vi "getData.vi"() -> ()   [LabVIEW 2014]
uses:
  <vilib>/FPGAPlugInAG/cRIO-9066/niLvFpga_Open_cRIO-9066.vi
  <vilib>/rvi/errors/niLvFpgaMergeErrorWithErrorCode.vi
  <vilib>/Utility/file.llb/Write To Spreadsheet File (DBL).vi
  <vilib>/FPGAPlugInAG/cRIO-9066/niLvFpga_Close_cRIO-9066.vi
  <vilib>/rvi/interface/nirviOpenFPGA/nirviOpenFPGA.xnode
  FPGA Bitfiles/forcecontroledu_FPGATarget_impElbow_wp9Tcc+MyeY.lvbitx
  FPGA VIs/imp_Elbow.vi
  <vilib>/rvi/interface/nirviMethod/nirviMethod.xnode
  <vilib>/rvi/interface/nirviCloseFPGA/nirviCloseFPGA.xnode
  <vilib>/FPGAPlugInAG/cRIO-9066/niLvFpga_ReadFifo_cRIO-9066.vi
panel:
  out "Loop count":i32=10000
  out "FIFO empty":bool
  out "sampling time":u32=10000
  out "message":string=" INSTRUCTIONS:\r\rNormal Use:  When using subVIs that incorporate the error in/error out (or error I/O) structure, place this handler where you want to inform the user of an error, typically at the end of the I/O data path, as the last action of the program.  If the error in error? is ERROR, the handler creates a message describing the error and its source.  If the type of dialog = 1 (default), the message is displayed to the user, who can only acknowedge it.  If the type = 2, the user can acknowledge the message or abort execution; aborting a program with active I/O is not recommended.  If the type = 0, no message is displayed; this is used to process the error programmatically, and the error out cluster elements are wired to individual terminals for that reason.  \r\rOther Use:\n\r\nlocal testing.  To test the error code of a subVI or function that does not have the error I/O structure, you can wire its error code and a source string to the local error code and error source inputs.  If error in error? indicates no error and error code is not equal to 0, the local code and source are substituted for the error in values, and error? is set TRUE (ERROR)."
  out "Elements Remaining":u32=10000
  in  "Number of samples":i32=10000
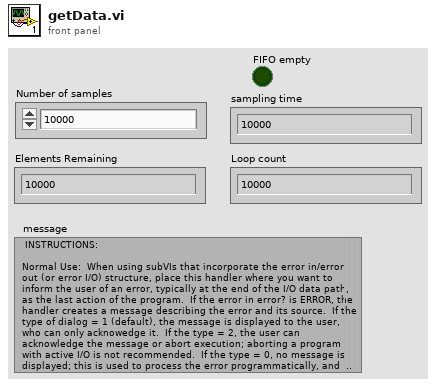
[diagram p1: front panel]
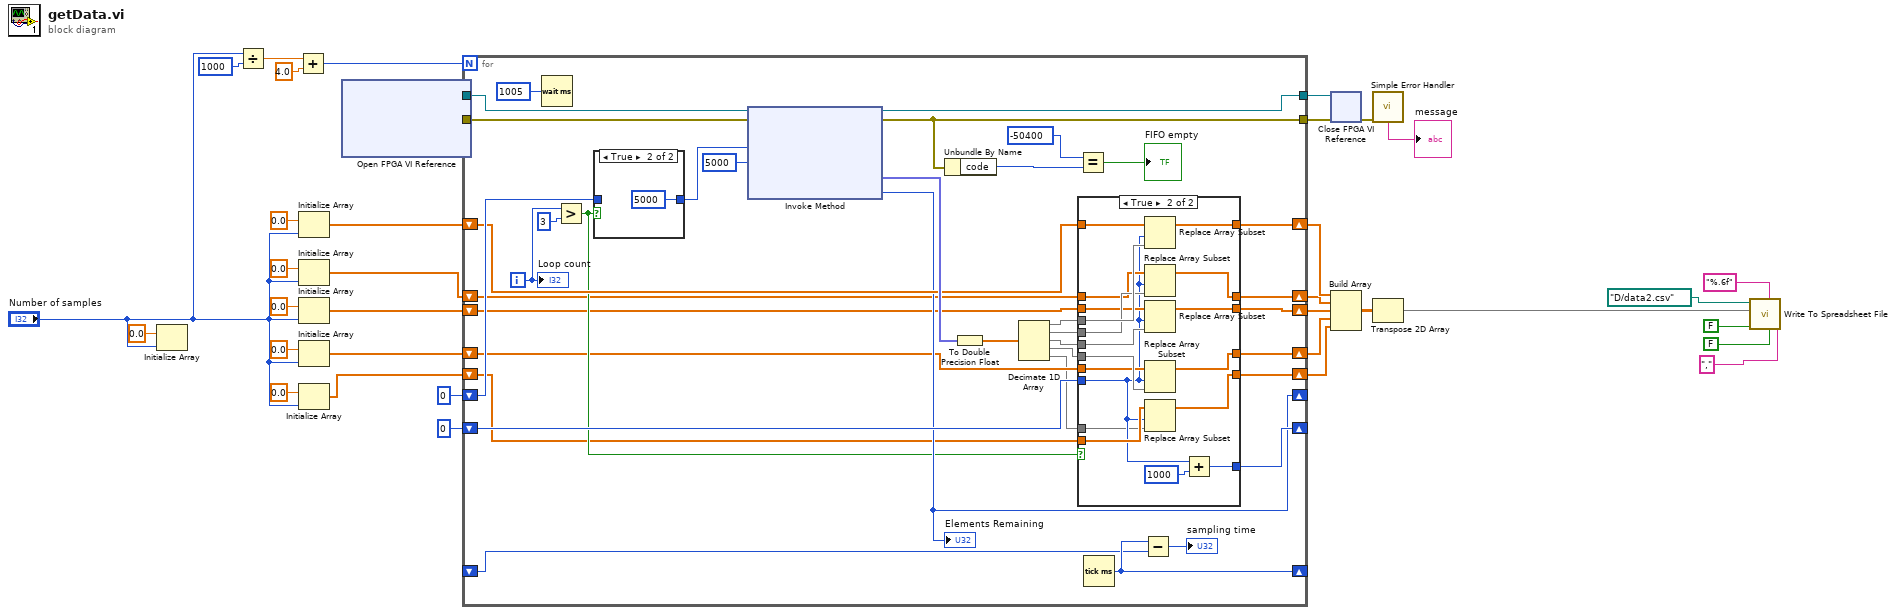
[diagram p0: block diagram]
diagram:
  n1 = Initialize Array(0.0 ("element"), "Number of samples") -> ()  [unwired: 1 out]
  n2 = Divide(x="Number of samples", y=1000) -> (x/y=w26:dbl)
  n3 = Add(x=w26, y=4.0) -> (x+y=w24:i32)
  n4 = Initialize Array(0.0 ("element"), "Number of samples") -> (w21:dbl[])
  n5 = Initialize Array(0.0 ("element"), "Number of samples") -> (w12:dbl[])
  n6 = Initialize Array(0.0 ("element"), "Number of samples") -> (w10:dbl[])
  n7 = Initialize Array(0.0 ("element"), "Number of samples") -> (w5:dbl[])
  n8 = Initialize Array(0.0 ("element"), "Number of samples") -> (w2:dbl[])
  n9 = xnode "Open FPGA VI Reference"() -> ("FPGA VI Reference Out"=w34:refnum<k20>, "error out"=w22:errorcluster)  [unwired: 2 in]
  n10 = for {
    N: w24 -> [_]
    tunnel: w34 -> [w71]
    tunnel: [w73] -> w36
    tunnel: [w54] -> w35
    tunnel: w22 -> [w70]
    shift-right: [w63] -> w20
    shift-left: w21 -> [w66]
    shift-right: [w64] -> _
    shift-left: 0 ("y") -> [w65]
    shift-right: [w61] -> _
    shift-left: u32 0 ("y") -> [w68]
    shift-right: [w62] -> _
    shift-left: _ -> [w60]
    shift-right: [w46] -> w9
    shift-left: w12 -> [w47]
    shift-right: [w43] -> w8
    shift-left: w10 -> [w44]
    shift-right: [w40] -> w4
    shift-left: w5 -> [w41]
    shift-right: [w37] -> w1
    shift-left: w2 -> [w39]
    i -> [w52]
    n11 = Wait (ms)(milliseconds to wait=u32 1005 ("millisecond multiple")) -> ()  [unwired: 1 out]
    n12 = Greater?(x=w52, y=3) -> (0:w57:bool)
    n13 = case shown="True" w57 {
      tunnel: w68 -> [w98 _]
      tunnel: [w98 u32 5000 ("y")] -> w67
      frame False {
      }
      frame True {
      }
    }
    n14 = xnode "Invoke Method"("FPGA VI Reference In"=w71, "error in"=w70, "Number of Elements"=w67, "Timeout (ms)"=5000) -> ("FPGA VI Reference Out"=w73:refnum<k20>, "error out"=w54:errorcluster, "Data"=w72:fxp<+/-,39,15>[], "Elements Remaining"=w61:u32)
    "Elements Remaining" <- w61
    n15 = Unbundle By Name(w54) -> ("code"=w53:i32)
    n16 = To Double Precision Float(number=w72) -> (double precision float=w50:dbl[])
    n17 = Decimate 1D Array(w50) -> (w49:dbl[], w48:dbl[], w45:dbl[], w42:dbl[], w38:dbl[])
    n18 = Equal?(x=-50400 ("y"), y=w53) -> (x = y?=→"FIFO empty":bool)
    n19 = case shown="True" w57 {
      tunnel: w66 -> [w78 w97]
      tunnel: w49 -> [_ w96]
      tunnel: w65 -> [w79 w82]
      tunnel: [w79 w94] -> w64
      tunnel: [w78 w93] -> w63
      tunnel: w48 -> [_ w92]
      tunnel: w47 -> [w77 w91]
      tunnel: [w77 w90] -> w46
      tunnel: w45 -> [_ w89]
      tunnel: w44 -> [w76 w88]
      tunnel: [w76 w87] -> w43
      tunnel: w42 -> [_ w86]
      tunnel: w41 -> [w75 w85]
      tunnel: [w75 w84] -> w40
      tunnel: w39 -> [w74 w83]
      tunnel: w38 -> [_ w81]
      tunnel: [w74 w80] -> w37
      frame False {
      }
      frame True {
        n20 = Replace Array Subset(array=w97, new element=w96, index=w82) -> (w93:dbl[])
        n21 = Replace Array Subset(array=w91, new element=w92, index=w82) -> (w90:dbl[])
        n22 = Replace Array Subset(array=w88, new element=w89, index=w82) -> (w87:dbl[])
        n23 = Replace Array Subset(array=w85, new element=w86, index=w82) -> (w84:dbl[])
        n24 = Replace Array Subset(array=w83, new element=w81, index=w82) -> (w80:dbl[])
        n25 = Add(x=w82, y=1000) -> (x+y=w94:i32)
      }
    }
    n26 = Tick Count (ms)() -> (millisecond timer value=w62:u32)
    n27 = Subtract(x=w62, y=w60) -> (x-y=→"sampling time":u32)
    "Loop count" <- w52
  }
  n28 = xnode "Close FPGA VI Reference"("FPGA VI Reference In"=w36, "error in"=w35) -> ("error out"=w17:errorcluster)
  n29 = Build Array(w20, w9, w8, w4, w1) -> (w19:dbl[][])
  n30 = call <vilib>:"Simple Error Handler.vi"("error in (no error)"=w17) -> ("message"=→"message":string)  [unwired: 4 in, 4 out]
  n31 = Transpose 2D Array(2D array=w19) -> (transposed array=w29:dbl[][])
  n32 = call-poly <vilib>:"Write To Spreadsheet File.vi"("delimiter (\\t)"="," ("delimiter (\\t)"), "transpose? (no:F)"=FALSE, "format (%.3f)"="%.6f" ("format (%d)"), "append to file? (new file:F)"=FALSE, "2D data"=w29, "file path (dialog if empty)"=path "D:/data2.csv") -> ()  [unwired: 2 in, 1 out]
